vi "Set Local Destination Path.vi"(8 "error in (no error)":errorcluster, 10 "Local destination path":path, 11 "NI_AB_API_DSDIST in":refnum<class "NI_AB_API_DSDIST.lvclass">) -> (0 "error out":errorcluster, 3 "NI_AB_API_DSDIST out":refnum<class "NI_AB_API_DSDIST.lvclass">)   [LabVIEW 2020, in "NI_AB_API_DSDIST.lvclass"]
uses:
  <vilib>/AppBuilder/AB_API/DSDIST/NI_AB_API_DSDIST.lvclass
  <vilib>/AppBuilder/AB_API/DSDIST/NI_AB_API_DSDIST.lvclass/NI_AB_API_DSDIST.ctl
  <vilib>/AppBuilder/AB_API/Build/NI_AB_API_Build.lvclass
  <vilib>/AppBuilder/AB_Classes/Build/AB_Build.lvclass
  e:/builds/penguin/labview/branches/2020/dev/dist/vi.lib/AppBuilder/AB_API/SDIST/NI_AB_API_SDIST.lvclass
  e:/builds/penguin/labview/branches/2020/dev/dist/vi.lib/AppBuilder/AB_API/Build/NI_AB_API_Build.lvclass
  e:/builds/penguin/labview/branches/2020/dev/dist/vi.lib/AppBuilder/AB_API/DSDIST/NI_AB_API_DSDIST.lvclass
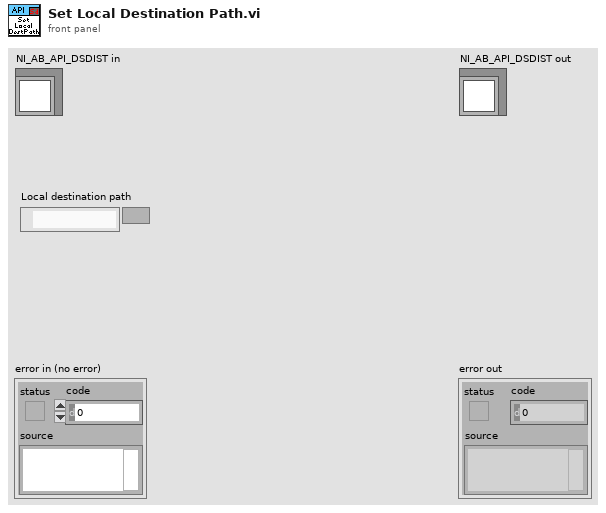
[diagram p1: front panel]
types:
  T1 = typedef "AB_Build.ctl" = cluster{"buildSpecName":string, "buildSpecDescription":string, "destinations":refnum<class "AB_Destination.lvclass">[], "exclusionOption":T2, "defaultLanguage":string, "supportedLanguages":string[], "excludedDirectories":path[], "buildContext":refnum<vi>, "buildObject":T3, "preview":bool, "programatic":bool, "progressBarEvents":T4, "userLog_Path":path, "preActionID":string, "preAction_Path":path, "postActionID":string, "postAction_Path":path, "eng_checkForBrokenVIs?":bool, "eng_verboseLinkerErrors?":bool, "localDest_Path":path, "targetDest_Path":path, "removeVIObject":u16, "cache":refnum<class "PreviewCache.lvclass">, "use cache":bool, "previewCache_ID":string, "buildCache_ID":string, "eng_TempLocalDest_Path":path, "eng_collectDependencies?":bool, "versionInfo":cluster{"buildVersion":cluster{"major":u16, "minor":u16, "patch":u16, "build":u16}, "autoIncrement":bool}, "eng_enableVIChecksums":bool}
  T2 = typedef "AB_Exclusion_Option.ctl" = cluster{"typedefs":bool, "polymorphicVIs":bool, "unusedLibraryItems":bool, "modifyLibraryFile":bool, "edit-timeDependencies":bool, "inlineVIs":bool, "dependent PPLs":bool, "dependent DLLs":bool}
  T3 = typedef "ItemRef.ctl" = u64
  T4 = typedef "provcom_ProgressBar_Events.ctl" = cluster{"newJob":refnum<user-event>, "newItem":refnum<user-event>, "errorMsg":T5, "cancel":refnum<user-event>}
  T5 = typedef "mxLvBuildError.ctl" = refnum<user-event>
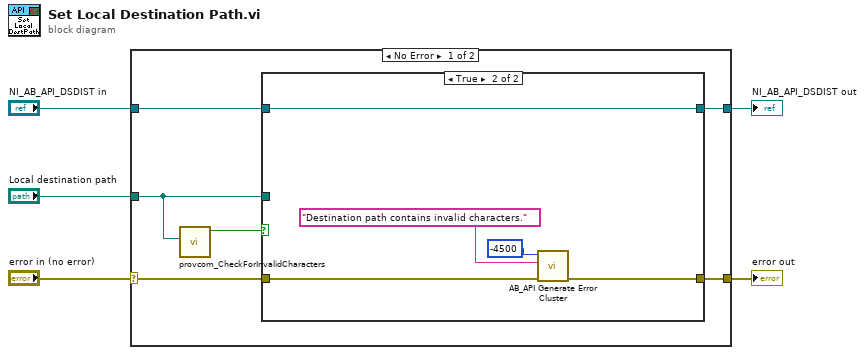
[diagram p0: block diagram]
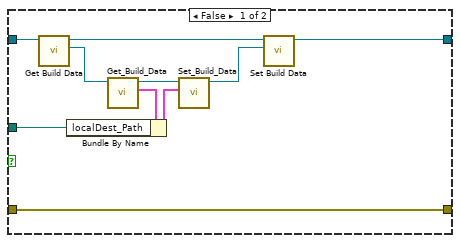
[diagram p2: hidden frame]
diagram:
  n1 = case shown="No Error" "error in (no error)" {
    selector: "error in (no error)" -> [w7 w28]
    tunnel: [w6 w28] -> w4
    tunnel: [w11 w27] -> w2
    tunnel: "NI_AB_API_DSDIST in" -> [w10 w27]
    tunnel: "Local destination path" -> [w9 _]
    frame No Error {
      n2 = call <resource>:"provcom_CheckForInvalidCharacters.vi"("NewPath"=w9) -> ("HasInvalidCharacters"=w8:bool)  [unwired: 2 in, 8 out]
      n3 = case shown="True" w8 {
        tunnel: [w21 w26] -> w11
        tunnel: w10 -> [w20 w26]
        tunnel: w9 -> [w13 _]
        tunnel: w7 -> [w12 w23]
        tunnel: [w12 w22] -> w6
        frame False {
          n4 = call <vilib>:"Get Build Data.vi"("NI_AB_API_Build in"=w20) -> ("AB_Build.lvclass"=w18:refnum<class "AB_Build.lvclass">, "NI_AB_API_Build out"=w19:refnum<class "NI_AB_API_DSDIST.lvclass">)  [unwired: 8 in, 1 out]
          n5 = call <vilib>:"Get_Build_Data.vi"("Class in"=w18) -> ("data"=w15:T1, "Class out"=w17:refnum<class "AB_Build.lvclass">)  [unwired: 8 in, 1 out]
          n6 = Bundle By Name(cluster=w15, "localDest_Path"=w13) -> (w14:T1)
          n7 = call <vilib>:"Set_Build_Data.vi"("data"=w14, "Class in"=w17) -> ("Class out"=w16:refnum<class "AB_Build.lvclass">)  [unwired: 8 in, 1 out]
          n8 = call <vilib>:"Set Build Data.vi"("AB_Build.lvclass"=w16, "NI_AB_API_Build in"=w19) -> ("NI_AB_API_Build out"=w21:refnum<class "NI_AB_API_DSDIST.lvclass">)  [unwired: 8 in, 1 out]
        }
        frame True {
          n9 = call <vilib>:"AB_API Generate Error Cluster.vi"("error in (no error)"=w23, "Additional Message"="Destination path contains invalid characters.", "Code"=-4500) -> ("error out"=w22:errorcluster)  [unwired: 1 in, 7 out]
        }
      }
    }
    frame Error {
    }
  }
  "error out" <- w4
  "NI_AB_API_DSDIST out" <- w2
